vi "Periodic Tasks.vi"(8 "error in (no error)":errorcluster) -> ()   [LabVIEW 2011]
doc: "This VI runs in parallel to other tasks. It can contain as many user-defined periodic loops as you need. These can carry out PID or other sorts of timed response."
uses:
  <vilib>/Rock Robotics/SystemInterfaces/Utilities/FPGA_UtilitiesLED State.ctl
  <vilib>/Rock Robotics/SystemInterfaces/Utilities/FPGA_UtilitiesLED Source.ctl
  <vilib>/Rock Robotics/WPI/Solenoid/WPI_SolenoidValue.ctl
  <vilib>/Rock Robotics/WPI/CAN/Jaguar/SubVIs/WPI_CANJaguar_StatusSelect.ctl
  <vilib>/Rock Robotics/WPI/Compressor/WPI_CompressorGetSetRefNum.vi
  Robot Global Data.vi
  <vilib>/Rock Robotics/WPI/Solenoid/Deprecated/WPI_SolenoidGetBool.vi
  <vilib>/Rock Robotics/WPI/Solenoid/WPI_SolenoidSetEnum.vi
panel:
  out "index":i32
  out "Target Locked":bool
  out "is not locked":bool
  out "is locked":bool
  out "Actual RPM":dbl
  out "Calculated RPM":dbl
  out "small error":bool
  out "poutput":dbl
  out "Distance from dash":dbl
  out "lr-v-out":dbl
  in  "Distance":dbl
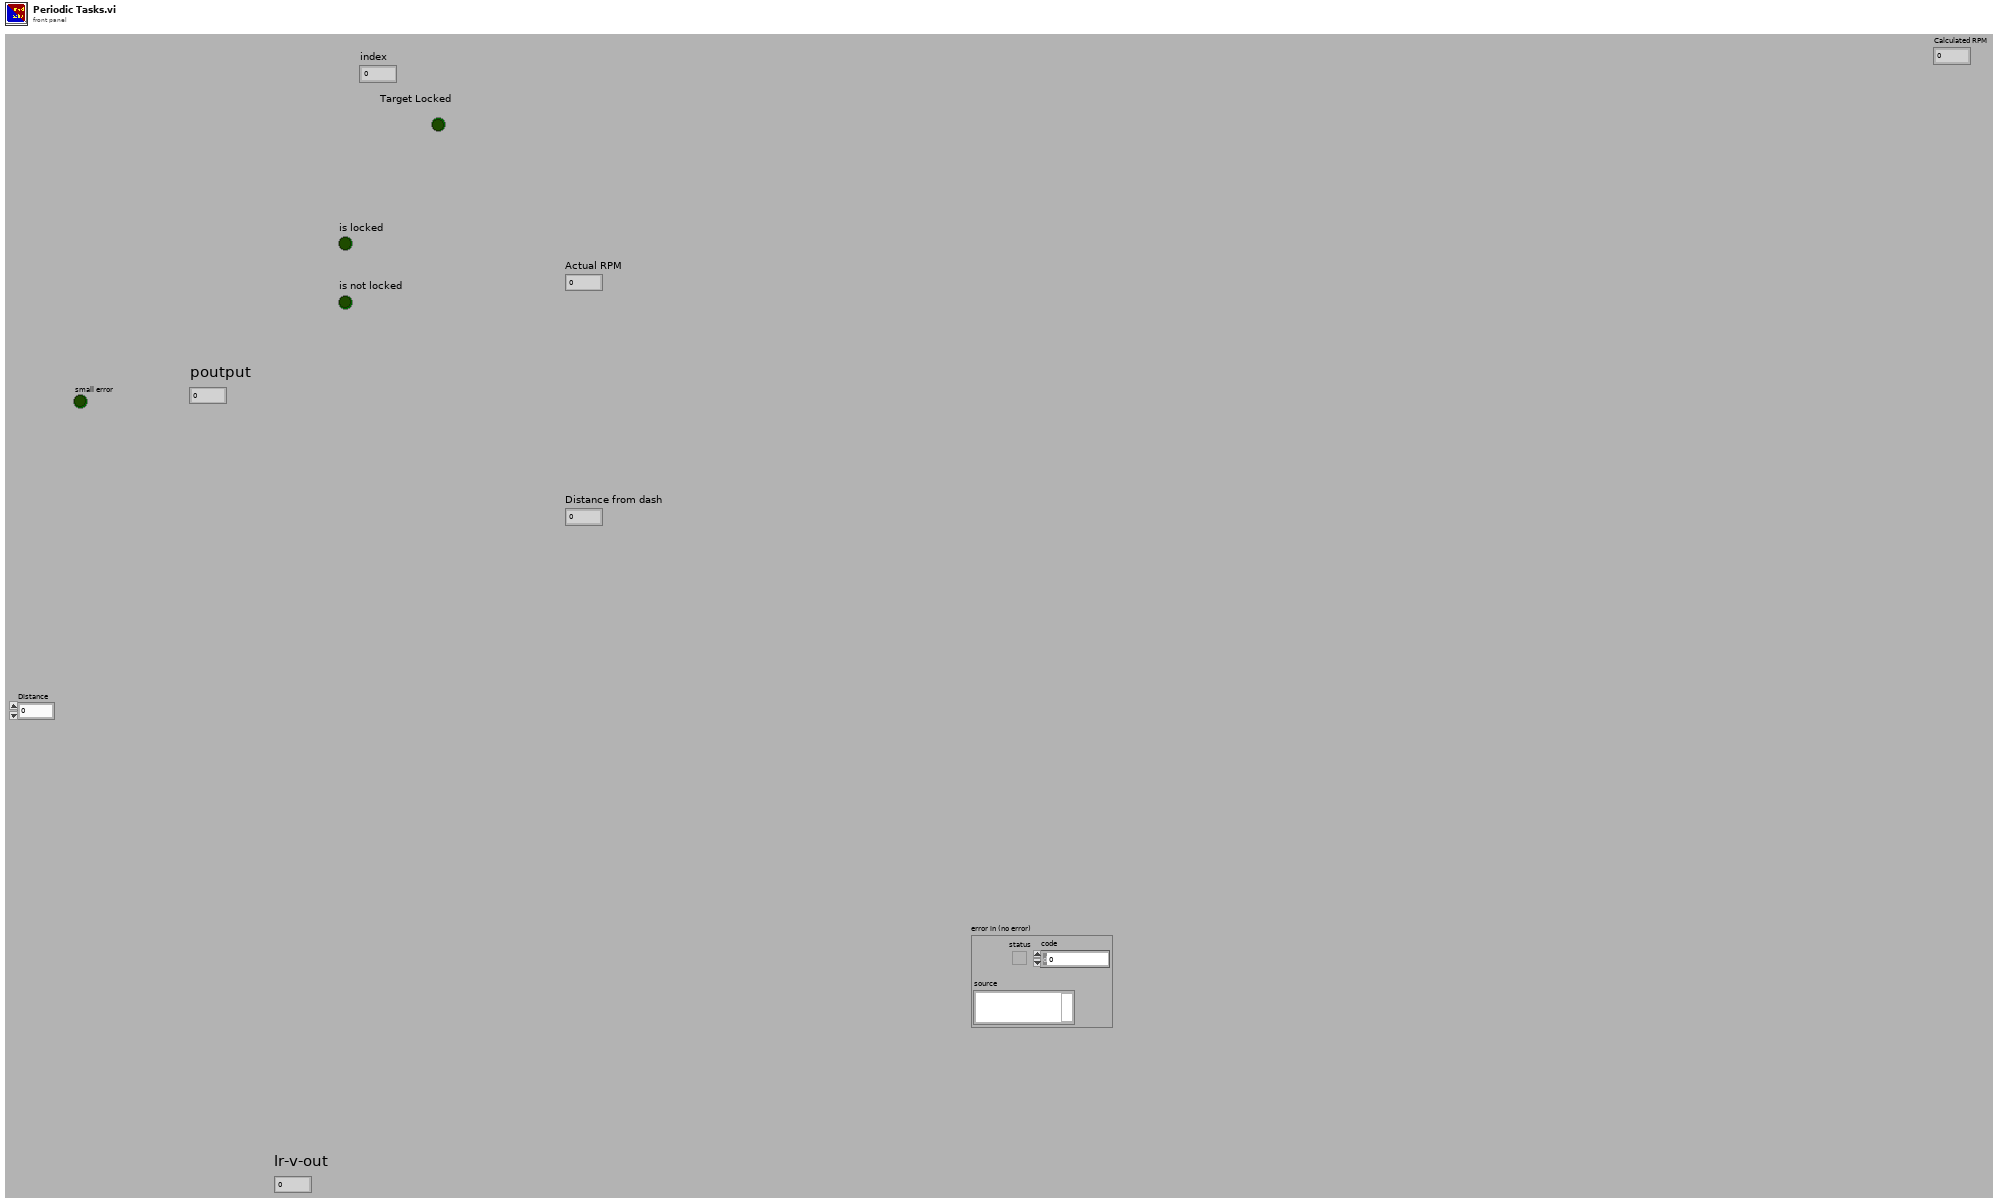
[diagram p1: front panel]
types:
  T1 = typedef "WPI_JoystickDevRef.ctl" = cluster{"Device":T2}
  T2 = typedef "WPI_JoystickDeviceEnum.ctl" = enum16{"USB 1", "USB 2", "USB 3", "USB 4", "Kinect 1", "Kinect 2"}
  T3 = typedef "WPI_JoystickButtonState.ctl" = cluster{"Button 1":bool, "Button 2":bool, "Button 3":bool, "Button 4":bool, "Button 5":bool, "Button 6":bool, "Button 7":bool, "Button 8":bool, "Button 9":bool, "Button 10":bool, "Button 11":bool, "Button 12":bool}
  T4 = cluster{"axis 1 (x)":dbl, "axis 2 (y)":dbl, "axis 3 (throttle)":dbl, "axis 4":dbl, "axis 5":dbl, "axis 6":dbl}
  T5 = typedef "WPI_CANJaguar_StatusSelect.ctl" = enum16{"Output Percent VBus", "Output Voltage", "Bus Voltage", "Current", "Temperature", "Position", "Speed", "Limit Switches", "Faults", "Fault Counters", "Power Cycle"}
  T6 = typedef "WPI_MotorControlDeviceRef.ctl" = cluster{"DeviceStatus":errorcluster, "Type":enum16{"PWM", "CAN"}, "PWM":cluster{"Digital Module":T7, "PWM Channel":T8, "DeadBand":T9}, "CAN":cluster{"Device Number":u8, "Control Mode":T10, "Semaphore":T11, "Max Vout":dbl}, "Invert":bool, "TransformRef":T12, "InvTransformRef":T12}
  T7 = typedef "FPGA_TypedefDigitalModule.ctl" = enum16{"Digital Module 1", "Digital Module 2"}
  T8 = typedef "FPGA_DIOPWMChannel.ctl" = enum8{"PWM 1", "PWM 2", "PWM 3", "PWM 4", "PWM 5", "PWM 6", "PWM 7", "PWM 8", "PWM 9", "PWM 10", "Invalid"}
  T9 = typedef "WPI_PWMDeadband.ctl" = cluster{"Name":string, "maxPositivePwm":i32, "minPositivePwm":i32, "centerPwm":i32, "maxNegativePwm":i32, "minNegativePwm":i32, "angularRange":u16}
  T10 = typedef "WPI_CANJaguar_ControlMode.ctl" = enum8{"Percent VBus", "Current", "Speed", "Position", "Voltage"}
  T11 = typedef "Semaphore RefNum" = refnum<k1>
  T12 = typedef "WPI_PWMTransform_ConPane.ctl" = refnum<vi>
  T13 = typedef "WPI_CANJaguar_Status.ctl" = cluster{"Output Percent VBus":dbl, "Output Voltage":dbl, "Bus Voltage":dbl, "Current":dbl, "Temperature":dbl, "Position":dbl, "Speed":dbl, "Limits":cluster{"Forward Limit":bool, "Reverse Limit":bool, "Forward Soft Limit":bool, "Reverse Soft Limit":bool, "Sticky Forward Limit":bool, "Sticky Reverse Limit":bool, "Sticky Forward Soft Limit":bool, "Sticky Reverse Soft Limit":bool}, "Faults":cluster{"Current Fault":bool, "Temperature Fault":bool, "Bus Voltage Fault":bool, "Gate Driver Fault":bool, "Comm Fault":bool}, "Fault Counters":cluster{"Current Faults":u8, "Temperature Faults":u8, "Bus Voltage Faults":u8, "Gate Driver Faults":u8, "Comm Faults":u8, "CAN Status":u8, "CAN RX Errors":u8, "CAN TX Errors":u8}, "Power Cycle":bool}
  T14 = typedef "FPGA_UtilitiesLED State.ctl" = enum16{"Off", "On", "Toggle"}
  T15 = typedef "FPGA_UtilitiesLED Source.ctl" = enum16{"User LED", "FPGA LED"}
  T16 = typedef "WPI_CompressorDevRef.ctl" = cluster{"DevStatus":errorcluster, "DigitalInputDevRef":T17, "RelayDevRef":T19}
  T17 = typedef "WPI_DigitalInputDevRef.ctl" = cluster{"DevStatus":errorcluster, "DIO Channel":T18, "Digital Module":T7}
  T18 = typedef "FPGA_DIOChannel.ctl" = enum8{"DIO 1", "DIO 2", "DIO 3", "DIO 4", "DIO 5", "DIO 6", "DIO 7", "DIO 8", "DIO 9", "DIO 10", "DIO 11", "DIO 12", "DIO 13", "DIO 14", "Invalid"}
  T19 = typedef "WPI_RelayDevRef.ctl" = cluster{"DevStatus":errorcluster, "Relay Channel":T20, "Digital Module":T7, "Relay Direction":T21}
  T20 = typedef "FPGA_DIORelayChannel.ctl" = enum8{"Relay 1", "Relay 2", "Relay 3", "Relay 4", "Relay 5", "Relay 6", "Relay 7", "Relay 8", "Invalid"}
  T21 = typedef "WPI_RelayDirection.ctl" = enum16{"Both directions", "Forward only", "Reverse only"}
  T22 = typedef "WPI_DigitalOutputDevRef.ctl" = cluster{"Digital Module":T7, "DIO Channel":T18, "DevStatus":errorcluster}
  T23 = cluster{"Selected Distance":dbl, "Calculated RPM":dbl, "Actual RPM":dbl, "Target Locked":bool}
  T24 = typedef "WPI_SolenoidValue.ctl" = enum16{"Off", "On", "Forward", "Reverse"}
  T25 = typedef "WPI_SolenoidDevRef.ctl" = cluster{"DevStatus":errorcluster, "Solenoid Module":T26, "Forward Solenoid Channel":T27, "Reverse Solenoid Channel":T27}
  T26 = typedef "FPGA_TypedefSolenoidModule.ctl" = enum16{"Solenoid Module 1", "Solenoid Module 2"}
  T27 = typedef "WPI_SolenoidChannel.ctl" = enum8{"Solenoid 1", "Solenoid 2", "Solenoid 3", "Solenoid 4", "Solenoid 5", "Solenoid 6", "Solenoid 7", "Solenoid 8", "Invalid"}
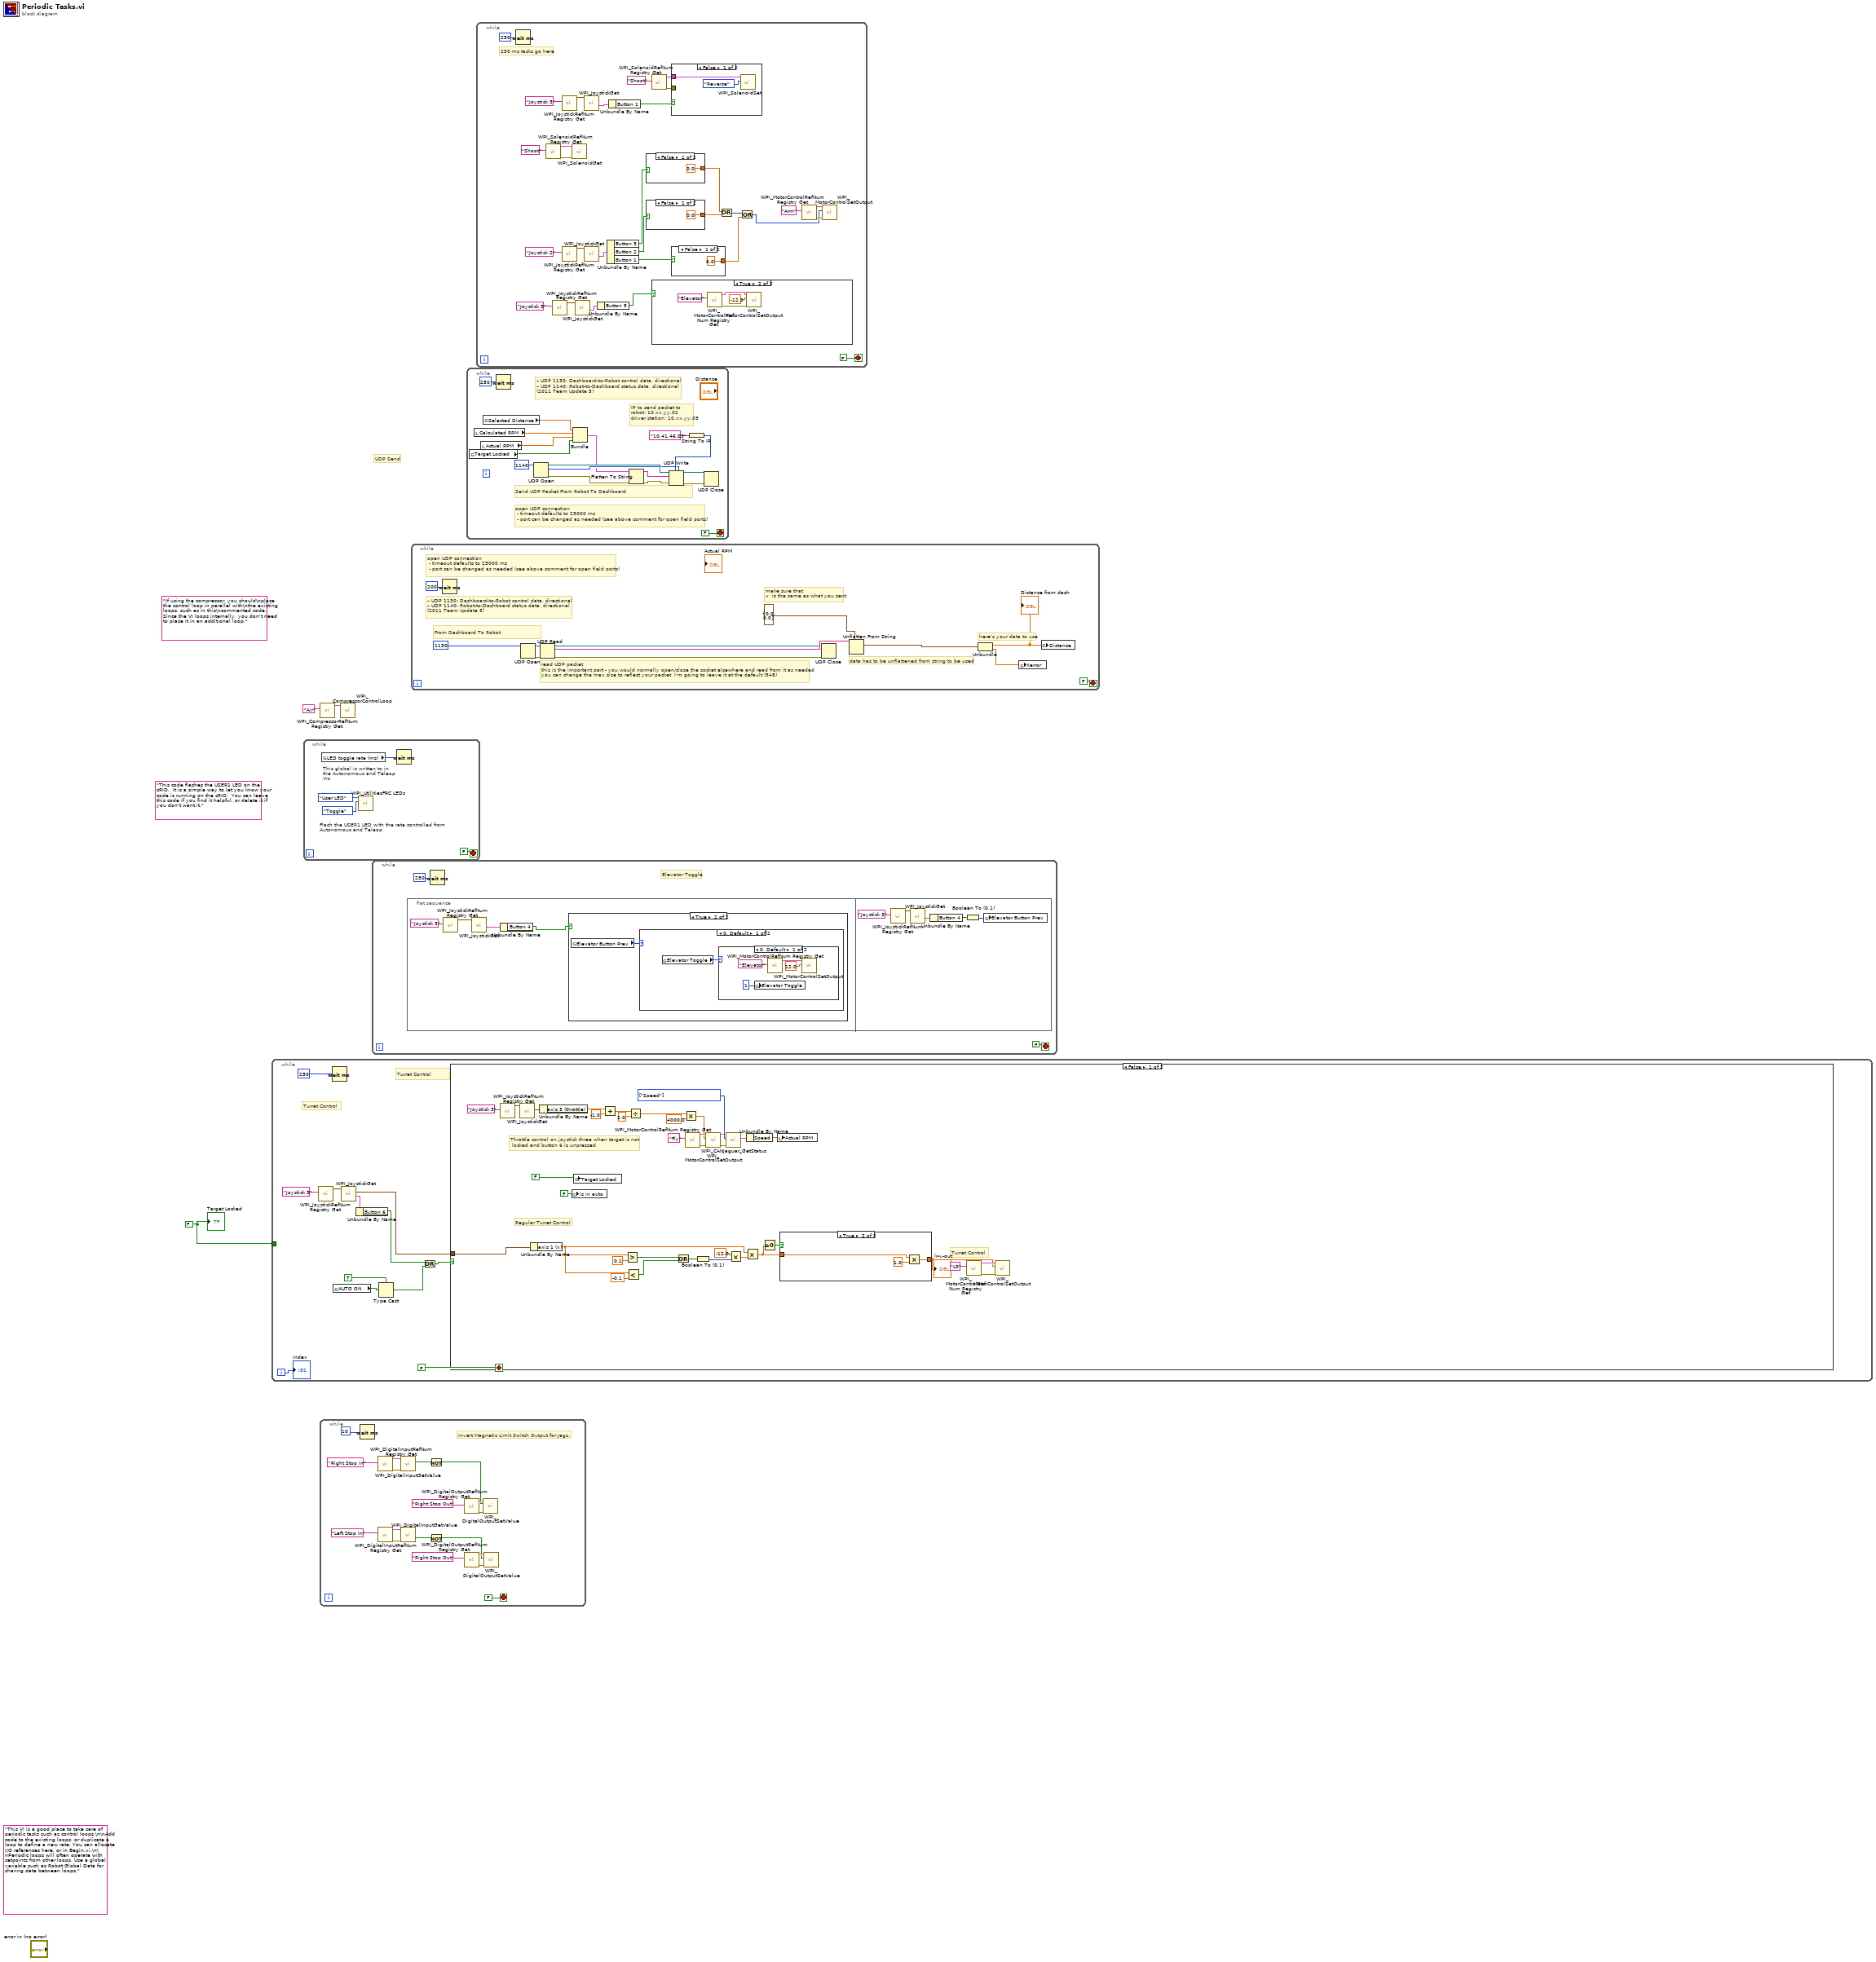
[diagram p0: block diagram]
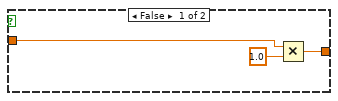
[diagram p2: hidden frame]
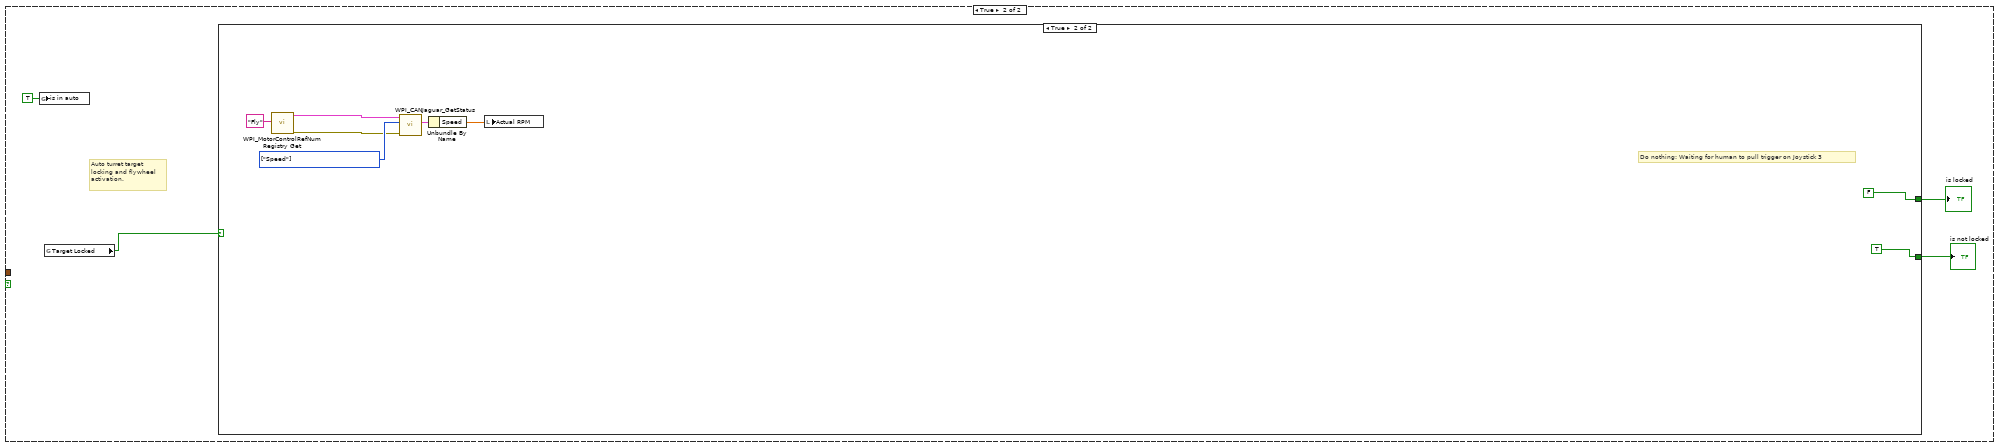
[diagram p3: hidden frame]
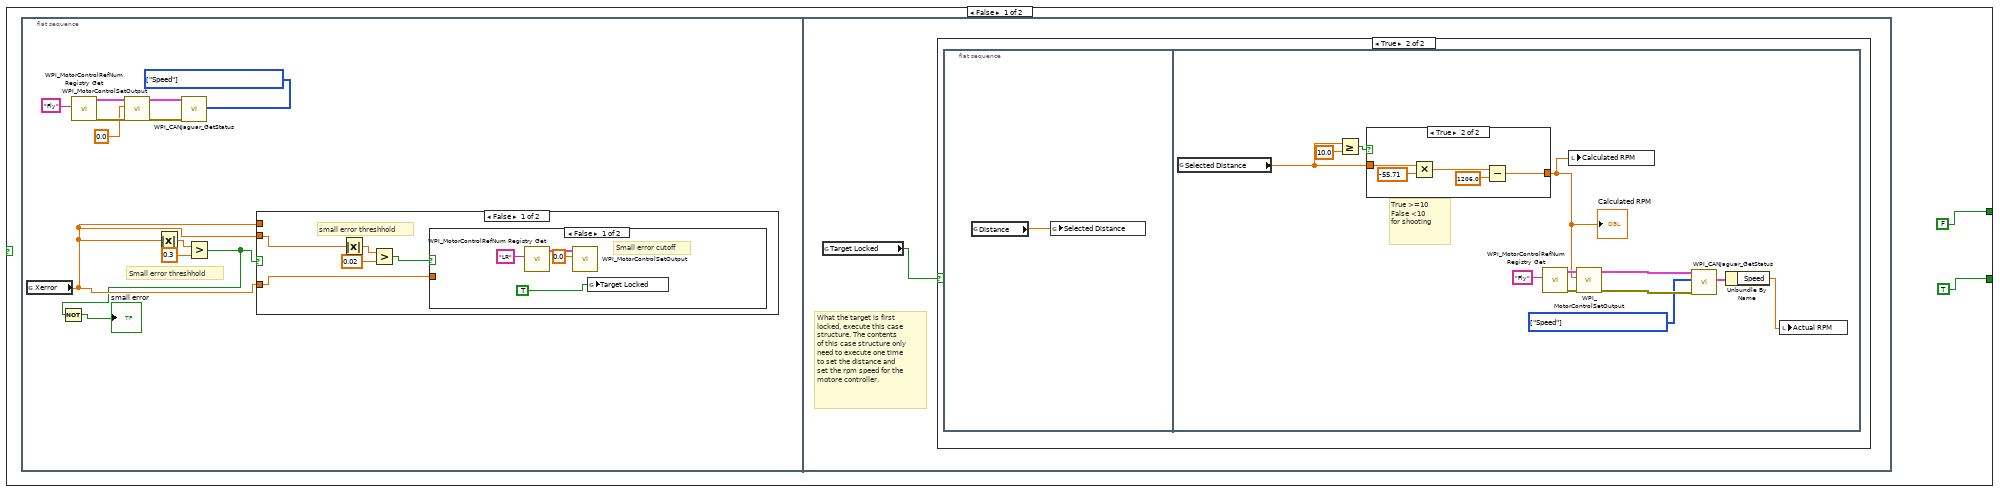
[diagram p4: hidden frame]
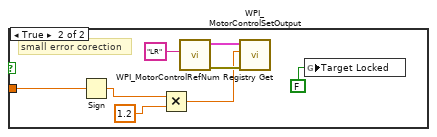
[diagram p5: hidden frame]
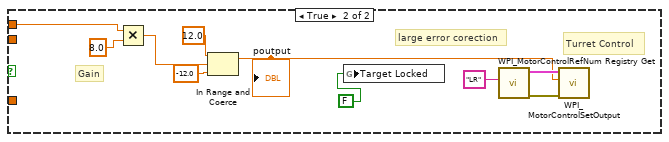
[diagram p6: hidden frame]
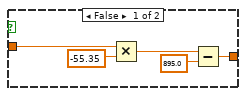
[diagram p8: hidden frame]
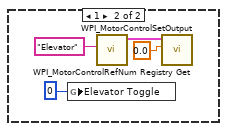
[diagram p10: hidden frame]
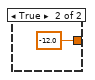
[diagram p12: hidden frame]
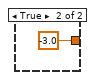
[diagram p13: hidden frame]
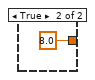
[diagram p14: hidden frame]
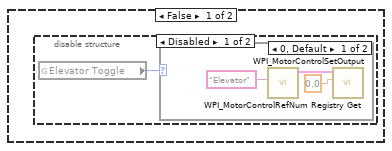
[diagram p15: hidden frame]
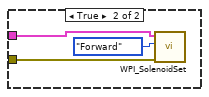
[diagram p18: hidden frame]
diagram:
  w3 = FALSE ("Target Locked")
  (unwired) "This VI is a good place to take care of periodic tasks such as control loops.\n\nAdd code to the existing loops, or duplicate a loop to define a new rate. You can allocate I/O references here, or in Begin.vi.\n\nPeriodic loops will often operate with setpoints from other loops. Use a global variable such as Robot Global Data for sharing data between loops."
  (unwired) "If using the compressor, you should\nplace the control loop in parallel with\nthe existing loops, such as in this\ncommented code. Since the VI loops internally, you don't need to place it in an additional loop."
  (unwired) "This code flashes the USER1 LED on the cRIO.  It is a simple way to let you know your code is running on the cRIO.  You can leave this code if you find it helpful, or delete it if you don't want it."
  # "UDP Send"
  n1 = while {
    tunnel: w3 -> [_]
    i -> [w10]
    stop <- FALSE stop-if-true
    # "Turret Control"
    # "Turret Control"
    n2 = call <vilib>:"WPI_JoystickRefNum Registry Get.vi"("refnum name"="Joystick 3") -> ("JoystickDevRef"=w13:T1)  [unwired: 9 in, 1 out]
    n3 = Wait (ms)(milliseconds to wait=u32 250) -> ()  [unwired: 1 out]
    n4 = global read "Robot Global Data.vi" "AUTO ON"() -> (w6:bool)
    n5 = call <vilib>:"WPI_JoystickGet.vi"("JoystickDevRef"=w13) -> ("Buttons"=w9:T3, "Axes"=w12:T4)  [unwired: 4 in, 1 out]
    n6 = Unbundle By Name(w9) -> ("Button 6"=w8:bool)
    n7 = Type Cast(type=TRUE, x=w6) -> (*(type *) &x=w4:bool)
    n8 = Or(x=w8, y=w4) -> (x .or. y?=w7:bool)
    n9 = case shown="False" w7 {
      tunnel: w12 -> [w47 _]
      frame False {
        w30 = T5[] [enum."Speed"] items=["Output Percent VBus", "Output Voltage", "Bus Voltage", "Current", "Temperature", "Position", "Speed", "Limit Switches", "Faults", "Fault Counters", "Power Cycle"] ("Status Select")
        # "Throttle control on joystick three when target is not\n locked and button 6 is unpressed"
        # "Regular Turret Control"
        # "Turret Control"
        n10 = call <vilib>:"WPI_JoystickRefNum Registry Get.vi"("refnum name"="Joystick 3") -> ("JoystickDevRef"=w26:T1)  [unwired: 9 in, 1 out]
        n11 = call <vilib>:"WPI_JoystickGet.vi"("JoystickDevRef"=w26) -> ("Axes"=w27:T4)  [unwired: 4 in, 2 out]
        n12 = Unbundle By Name(w47) -> ("axis 1 (x)"=w39:dbl)
        n13 = Unbundle By Name(w27) -> ("axis 3 (throttle)"=w24:dbl)
        n14 = global write "Robot Global Data.vi" "is in auto"(FALSE ("is in auto")) -> ()
        n15 = global write "Robot Global Data.vi" "Target Locked"(FALSE ("Target Locked")) -> ()
        n16 = Add(x=w24, y=-1.0) -> (x+y=w22:dbl)
        n17 = Greater?(x=w39, y=0.1) -> (0:w44:bool)
        n18 = Less?(x=w39, y=-0.1) -> (x < y?=w43:bool)
        n19 = Divide(x=w22, y=2.0) -> (x/y=w16:dbl)
        n20 = Or(x=w44, y=w43) -> (x .or. y?=w42:bool)
        n21 = Multiply(x=w16, y=4000.0) -> (x*y=w19:dbl)
        n22 = call <vilib>:"WPI_MotorControlRefNum Registry Get.vi"("refnum name"="Fly") -> ("error out"=w31:errorcluster, "MotorControlDevRef"=w32:T6)  [unwired: 9 in]
        n23 = Boolean To (0,1)(Boolean=w42) -> (0, 1=w41:i16)
        n24 = call <vilib>:"WPI_MotorControlSetOutput.vi"("error in (no error)"=w31, "Output"=w19, "MotorControlDevRef"=w32) -> ("error out"=w28:errorcluster, "MotorControlDevRef"=w29:T6)  [unwired: 7 in]
        n25 = call <vilib>:"WPI_CANJaguar_GetStatus.vi"("error in (no error)"=w28, "Status Select"=w30, "CAN Jaguar Ref"=w29) -> ("Status"=w18:T13)  [unwired: 6 in, 2 out]
        n26 = Multiply(x=-12.0, y=w41) -> (x*y=w40:dbl)
        n27 = Multiply(x=w39, y=w40) -> (x*y=w37:dbl)
        n28 = Unbundle By Name(w18) -> ("Speed"=w17:dbl)
        n29 = Greater Or Equal To 0?(x=w37) -> (x >= 0?=w38:bool)
        n30 = local write "Actual RPM"(w17) -> ()
        n31 = case shown="True" w38 {
          tunnel: w37 -> [w54 w57]
          tunnel: [w53 w56] -> w36
          frame False {
            n32 = Multiply(x=w54, y=1.0) -> (x*y=w53:dbl)
          }
          frame True {
            n33 = Multiply(x=w57, y=1.0) -> (x*y=w56:dbl)
          }
        }
        "lr-v-out" <- w36
        n34 = call <vilib>:"WPI_MotorControlRefNum Registry Get.vi"("refnum name"="LR") -> ("error out"=w50:errorcluster, "MotorControlDevRef"=w51:T6)  [unwired: 9 in]
        n35 = call <vilib>:"WPI_MotorControlSetOutput.vi"("error in (no error)"=w50, "Output"=w36, "MotorControlDevRef"=w51) -> ()  [unwired: 7 in, 2 out]
      }
      frame True {
        # "Auto turret target\nlocking and flywheel\nactivation."
        n36 = global write "Robot Global Data.vi" "is in auto"(TRUE ("is in auto")) -> ()
        n37 = global read "Robot Global Data.vi" "Target Locked"() -> (w58:bool)
        n38 = case shown="True" w58 {
          tunnel: [FALSE FALSE] -> w60
          tunnel: [TRUE TRUE] -> w59
          frame False {
            n39 = flat-sequence {
              frame #0 {
                w72 = T5[] [enum."Speed"] items=["Output Percent VBus", "Output Voltage", "Bus Voltage", "Current", "Temperature", "Position", "Speed", "Limit Switches", "Faults", "Fault Counters", "Power Cycle"] ("Status Select")
                # "Small error threshhold"
                n40 = global read "Robot Global Data.vi" "Xerror"() -> (w68:dbl)
                n41 = call <vilib>:"WPI_MotorControlRefNum Registry Get.vi"("refnum name"="Fly") -> ("error out"=w73:errorcluster, "MotorControlDevRef"=w74:T6)  [unwired: 9 in]
                n42 = call <vilib>:"WPI_MotorControlSetOutput.vi"("error in (no error)"=w73, "Output"=0.0, "MotorControlDevRef"=w74) -> ("error out"=w69:errorcluster, "MotorControlDevRef"=w70:T6)  [unwired: 7 in]
                n43 = Absolute Value(x=w68) -> (abs(x)=w64:dbl)
                n44 = call <vilib>:"WPI_CANJaguar_GetStatus.vi"("error in (no error)"=w69, "Status Select"=w72, "CAN Jaguar Ref"=w70) -> ()  [unwired: 6 in, 3 out]
                n45 = Greater?(x=w64, y=0.3) -> (0:w67:bool)
                n46 = Not(x=w67) -> (.not. x?=→"small error":bool)
                n47 = case shown="False" w67 {
                  tunnel: w68 -> [_ w98]
                  tunnel: w68 -> [w80 _]
                  tunnel: w68 -> [w77 _]
                  frame False {
                    # "small error threshhold"
                    n48 = Absolute Value(x=w77) -> (abs(x)=w79:dbl)
                    n49 = Greater?(x=w79, y=0.02) -> (0:w76:bool)
                    n50 = case shown="False" w76 {
                      tunnel: w80 -> [_ w89]
                      frame False {
                        # "Small error cutoff"
                        n51 = call <vilib>:"WPI_MotorControlRefNum Registry Get.vi"("refnum name"="LR") -> ("MotorControlDevRef"=w84:T6)  [unwired: 9 in, 1 out]
                        n52 = call <vilib>:"WPI_MotorControlSetOutput.vi"("Output"=0.0, "MotorControlDevRef"=w84) -> ()  [unwired: 8 in, 2 out]
                        n53 = global write "Robot Global Data.vi" "Target Locked"(TRUE ("Target Locked")) -> ()
                      }
                      frame True {
                        # "small error corection"
                        n54 = Sign(1:w89) -> (0:w88:dbl)
                        n55 = Multiply(x=w88, y=1.2) -> (x*y=w87:dbl)
                        n56 = call <vilib>:"WPI_MotorControlRefNum Registry Get.vi"("refnum name"="LR") -> ("error out"=w91:errorcluster, "MotorControlDevRef"=w92:T6)  [unwired: 9 in]
                        n57 = call <vilib>:"WPI_MotorControlSetOutput.vi"("error in (no error)"=w91, "Output"=w87, "MotorControlDevRef"=w92) -> ()  [unwired: 7 in, 2 out]
                        n58 = global write "Robot Global Data.vi" "Target Locked"(FALSE ("Target Locked")) -> ()
                      }
                    }
                  }
                  frame True {
                    # "large error corection"
                    # "Gain"
                    # "Turret Control"
                    n59 = Multiply(x=w98, y=8.0) -> (x*y=w95:dbl)
                    n60 = In Range and Coerce(upper limit=12.0, x=w95, lower limit=-12.0) -> (coerced(x)=w97:dbl)  [unwired: 1 out]
                    "poutput" <- w97
                    n61 = global write "Robot Global Data.vi" "Target Locked"(FALSE ("Target Locked")) -> ()
                    n62 = call <vilib>:"WPI_MotorControlRefNum Registry Get.vi"("refnum name"="LR") -> ("error out"=w101:errorcluster, "MotorControlDevRef"=w102:T6)  [unwired: 9 in]
                    n63 = call <vilib>:"WPI_MotorControlSetOutput.vi"("error in (no error)"=w101, "Output"=w97, "MotorControlDevRef"=w102) -> ()  [unwired: 7 in, 2 out]
                  }
                }
              }
              frame #1 {
                # "What the target is first\nlocked, execute this case\nstructure. The contents\nof this case structure only\nneed to execute one time\nto set the distance and\nset the rpm speed for the\nmotore controller."
                n64 = global read "Robot Global Data.vi" "Target Locked"() -> (w103:bool)
                n65 = case shown="True" w103 {
                  frame False {
                  }
                  frame True {
                    n66 = flat-sequence {
                      frame #0 {
                        n67 = global read "Robot Global Data.vi" "Distance"() -> (w104:dbl)
                        n68 = global write "Robot Global Data.vi" "Selected Distance"(w104) -> ()
                      }
                      frame #1 {
                        w109 = T5[] [enum."Speed"] items=["Output Percent VBus", "Output Voltage", "Bus Voltage", "Current", "Temperature", "Position", "Speed", "Limit Switches", "Faults", "Fault Counters", "Power Cycle"] ("Status Select")
                        # "True >=10\nFalse <10\nfor shooting"
                        n69 = global read "Robot Global Data.vi" "Selected Distance"() -> (w107:dbl)
                        n70 = Greater Or Equal?(x=w107, y=10.0) -> (x >= y?=w112:bool)
                        n71 = case shown="True" w112 {
                          tunnel: w107 -> [w117 w122]
                          tunnel: [w121 w126] -> w106
                          frame False {
                            n72 = Multiply(x=w117, y=-55.35) -> (x*y=w119:dbl)
                            n73 = Subtract(x=w119, y=895.0) -> (x-y=w121:dbl)
                          }
                          frame True {
                            n74 = Multiply(x=w122, y=-55.71) -> (x*y=w124:dbl)
                            n75 = Subtract(x=w124, y=1206.0) -> (x-y=w126:dbl)
                          }
                        }
                        "Calculated RPM" <- w106
                        n76 = call <vilib>:"WPI_MotorControlRefNum Registry Get.vi"("refnum name"="Fly") -> ("error out"=w114:errorcluster, "MotorControlDevRef"=w115:T6)  [unwired: 9 in]
                        n77 = local write "Calculated RPM"(w106) -> ()
                        n78 = call <vilib>:"WPI_MotorControlSetOutput.vi"("error in (no error)"=w114, "Output"=w106, "MotorControlDevRef"=w115) -> ("error out"=w110:errorcluster, "MotorControlDevRef"=w111:T6)  [unwired: 7 in]
                        n79 = call <vilib>:"WPI_CANJaguar_GetStatus.vi"("error in (no error)"=w110, "Status Select"=w109, "CAN Jaguar Ref"=w111) -> ("Status"=w108:T13)  [unwired: 6 in, 2 out]
                        n80 = Unbundle By Name(w108) -> ("Speed"=w105:dbl)
                        n81 = local write "Actual RPM"(w105) -> ()
                      }
                    }
                  }
                }
              }
            }
          }
          frame True {
            w133 = T5[] [enum."Speed"] items=["Output Percent VBus", "Output Voltage", "Bus Voltage", "Current", "Temperature", "Position", "Speed", "Limit Switches", "Faults", "Fault Counters", "Power Cycle"] ("Status Select")
            # "Do nothing: Waiting for human to pull trigger on Joystick 3"
            n82 = call <vilib>:"WPI_MotorControlRefNum Registry Get.vi"("refnum name"="Fly") -> ("error out"=w129:errorcluster, "MotorControlDevRef"=w130:T6)  [unwired: 9 in]
            n83 = call <vilib>:"WPI_CANJaguar_GetStatus.vi"("error in (no error)"=w129, "Status Select"=w133, "CAN Jaguar Ref"=w130) -> ("Status"=w132:T13)  [unwired: 6 in, 2 out]
            n84 = Unbundle By Name(w132) -> ("Speed"=w131:dbl)
            n85 = local write "Actual RPM"(w131) -> ()
          }
        }
        "is locked" <- w60
        "is not locked" <- w59
      }
    }
    "index" <- w10
  }
  n86 = while {
    stop <- FALSE stop-if-true
    # "This global is written to in the Autonomous and Teleop VIs"
    # "Flash the USER1 LED with the rate controlled from Autonomous and Teleop"
    n87 = global read "Robot Global Data.vi" "LED toggle rate (ms)"() -> (w135:u32)
    n88 = call <vilib>:"WPI_UtilitiesFRC LEDs.vi"("State"=FPGA_UtilitiesLED_State."Toggle", "LED Type"=FPGA_UtilitiesLED_Source."User LED") -> ()  [unwired: 1 in, 9 out]
    n89 = Wait (ms)(milliseconds to wait=w135) -> ()  [unwired: 1 out]
  }
  n90 = call <vilib>:"WPI_CompressorRefNum Registry Get.vi"("refnum name"="Air") -> ("CompressorDevRef"=w2:T16)  [unwired: 9 in, 1 out]
  n91 = while {
    stop <- FALSE stop-if-true
    # "Invert Magnetic Limit Switch Output for Jags."
    n92 = Wait (ms)(milliseconds to wait=u32 10) -> ()  [unwired: 1 out]
    n93 = call <vilib>:"WPI_DigitalInputRefNum Registry Get.vi"("refnum name"="Right Stop In") -> ("error out"=w149:errorcluster, "DigitalInputDevRef"=w152:T17)  [unwired: 9 in]
    n94 = call <vilib>:"WPI_DigitalInputRefNum Registry Get.vi"("refnum name"="Left Stop In") -> ("error out"=w150:errorcluster, "DigitalInputDevRef"=w153:T17)  [unwired: 9 in]
    n95 = call <vilib>:"WPI_DigitalInputGetValue.vi"("error in (no error)"=w149, "DigitalInputDevRef"=w152) -> ("Value"=w140:bool)  [unwired: 7 in, 2 out]
    n96 = call <vilib>:"WPI_DigitalInputGetValue.vi"("error in (no error)"=w150, "DigitalInputDevRef"=w153) -> ("Value"=w142:bool)  [unwired: 7 in, 2 out]
    n97 = Not(x=w140) -> (.not. x?=w139:bool)
    n98 = Not(x=w142) -> (.not. x?=w141:bool)
    n99 = call <vilib>:"WPI_DigitalOutputRefNum Registry Get.vi"("refnum name"="Right Stop Out") -> ("error out"=w144:errorcluster, "DigitalOutputDevRef"=w143:T22)  [unwired: 9 in]
    n100 = call <vilib>:"WPI_DigitalOutputRefNum Registry Get.vi"("refnum name"="Right Stop Out") -> ("error out"=w146:errorcluster, "DigitalOutputDevRef"=w145:T22)  [unwired: 9 in]
    n101 = call <vilib>:"WPI_DigitalOutputSetValue.vi"("error in (no error)"=w144, "Value"=w139, "DigitalOutputDevRef"=w143) -> ()  [unwired: 7 in, 2 out]
    n102 = call <vilib>:"WPI_DigitalOutputSetValue.vi"("error in (no error)"=w146, "Value"=w141, "DigitalOutputDevRef"=w145) -> ()  [unwired: 7 in, 2 out]
  }
  n103 = call <vilib>:"WPI_CompressorControlLoop.vi"("CompressorDevRef"=w2) -> ()  [unwired: 11 in]
  n104 = while {
    stop <- FALSE stop-if-true
    # "Elevator Toggle"
    n105 = flat-sequence {
      frame #0 {
        n106 = call <vilib>:"WPI_JoystickRefNum Registry Get.vi"("refnum name"="Joystick 3") -> ("JoystickDevRef"=w161:T1)  [unwired: 9 in, 1 out]
        n107 = call <vilib>:"WPI_JoystickGet.vi"("JoystickDevRef"=w161) -> ("Buttons"=w160:T3)  [unwired: 4 in, 2 out]
        n108 = Unbundle By Name(w160) -> ("Button 4"=w159:bool)
        n109 = case shown="True" w159 {
          frame False {
          }
          frame True {
            n110 = global read "Robot Global Data.vi" "Elevator Button Prev"() -> (w163:u8)
            n111 = case shown="0, Default" w163 {
              frame 0, Default {
                n112 = global read "Robot Global Data.vi" "Elevator Toggle"() -> (w164:u8)
                n113 = case shown="0, Default" w164 {
                  frame 0, Default {
                    n114 = global write "Robot Global Data.vi" "Elevator Toggle"(u8 1 ("Elevator Toggle")) -> ()
                    n115 = call <vilib>:"WPI_MotorControlRefNum Registry Get.vi"("refnum name"="Elevator") -> ("MotorControlDevRef"=w167:T6)  [unwired: 9 in, 1 out]
                    n116 = call <vilib>:"WPI_MotorControlSetOutput.vi"("Output"=12.0 ("y"), "MotorControlDevRef"=w167) -> ()  [unwired: 8 in, 2 out]
                  }
                  frame 1 {
                    n117 = global write "Robot Global Data.vi" "Elevator Toggle"(u8 0 ("Elevator Toggle")) -> ()
                    n118 = call <vilib>:"WPI_MotorControlRefNum Registry Get.vi"("refnum name"="Elevator") -> ("MotorControlDevRef"=w170:T6)  [unwired: 9 in, 1 out]
                    n119 = call <vilib>:"WPI_MotorControlSetOutput.vi"("Output"=0.0 ("y"), "MotorControlDevRef"=w170) -> ()  [unwired: 8 in, 2 out]
                  }
                }
              }
              frame 1 {
              }
            }
          }
        }
      }
      frame #1 {
        n120 = call <vilib>:"WPI_JoystickRefNum Registry Get.vi"("refnum name"="Joystick 3") -> ("JoystickDevRef"=w176:T1)  [unwired: 9 in, 1 out]
        n121 = call <vilib>:"WPI_JoystickGet.vi"("JoystickDevRef"=w176) -> ("Buttons"=w177:T3)  [unwired: 4 in, 2 out]
        n122 = Unbundle By Name(w177) -> ("Button 4"=w174:bool)
        n123 = Boolean To (0,1)(Boolean=w174) -> (0, 1=w173:i16)
        n124 = global write "Robot Global Data.vi" "Elevator Button Prev"(w173) -> ()
      }
    }
    n125 = Wait (ms)(milliseconds to wait=u32 250) -> ()  [unwired: 1 out]
  }
  n126 = while {
    stop <- FALSE stop-if-true
    # "here's your data to use"
    # "make sure that\nv  is the same as what you sent"
    # "data has to be unflattened from string to be used"
    # "read UDP packet\nthis is the important part - you would normally open/close the socket elsewhere and read from it as needed\nyou can change the max size to reflect your packet, I'm going to leave it at the default (548)"
    # "open UDP connection\n - timeout defaults to 25000 ms\n - port can be changed as needed (see above comment for open field ports)"
    # "– UDP 1130: Dashboard-to-Robot control data, directional\n– UDP 1140: Robot-to-Dashboard status data, directional\n(2011 Team Update 5)"
    # "From Dashboard To Robot"
    n127 = Wait (ms)(milliseconds to wait=u32 200) -> ()  [unwired: 1 out]
    n128 = UDP Open(11:u16 1130 ("port")) -> (port=w188:refnum<k16>, 0:w187:errorcluster)  [unwired: 1 in, 4 out]
    n129 = UDP Read(connection ID=w188, 8:w187) -> (data out=w186:string, error out=w182:errorcluster, 3:w183:refnum<k16>)  [unwired: 4 out]
    n130 = UDP Close(connection ID=w183, 8:w182) -> ()  [unwired: 2 out]
    n131 = Unflatten From String(type=cluster{dbl, dbl} {0.0, 0.0}, binary string=w186) -> (value=w184:cluster{dbl, dbl})  [unwired: 1 in, 4 out]
    n132 = Unbundle(w184) -> (w179:dbl, w178:dbl)
    "Distance from dash" <- w179
    n133 = global write "Robot Global Data.vi" "Xerror"(w178) -> ()
    n134 = global write "Robot Global Data.vi" "Distance"(w179) -> ()
  }
  n135 = while {
    stop <- FALSE stop-if-true
    # "IP to send packet to \nrobot: 10.xx.yy.02\ndriver station: 10.xx.yy.09"
    # "open UDP connection\n - timeout defaults to 25000 ms\n - port can be changed as needed (see above comment for open field ports)"
    # "Send UDP Packet From Robot To Dashboard"
    # "– UDP 1130: Dashboard-to-Robot control data, directional\n– UDP 1140: Robot-to-Dashboard status data, directional\n(2011 Team Update 5)"
    n136 = global read "Robot Global Data.vi" "Target Locked"() -> (w190:bool)
    n137 = local read "Calculated RPM"() -> (w194:dbl)
    n138 = local read "Actual RPM"() -> (w193:dbl)
    n139 = global read "Robot Global Data.vi" "Selected Distance"() -> (w195:dbl)
    n140 = Wait (ms)(milliseconds to wait=u32 250) -> ()  [unwired: 1 out]
    n141 = UDP Open(11:u16 1140 ("port")) -> (port=w199:refnum<k16>, 0:w197:errorcluster, 2:w198:u16)  [unwired: 1 in, 3 out]
    n142 = Bundle("Selected Distance"=w195, "Calculated RPM"=w194, "Actual RPM"=w193, "Target Locked"=w190) -> (w192:T23)  [unwired: 1 in]
    n143 = Flatten To String(anything=w192, error in (no error)=w197) -> (data string=w203:string, error out=w204:errorcluster)  [unwired: 3 out]
    n144 = String To IP(1:"10.41.46.09") -> (0:w205:u32)
    n145 = UDP Write(address=w205, port or service name=w198, connection ID=w199, data in=w203, 8:w204) -> (error out=w201:errorcluster, 3:w202:refnum<k16>)  [unwired: 1 out]
    n146 = UDP Close(connection ID=w202, 8:w201) -> ()  [unwired: 2 out]
  }
  n147 = while {
    stop <- FALSE stop-if-true
    # "250 ms tasks go here"
    n148 = Wait (ms)(milliseconds to wait=u32 250) -> ()  [unwired: 1 out]
    n149 = call <vilib>:"WPI_SolenoidRefNum Registry Get.vi"("refnum name"="Shoot") -> ("error out"=w231:errorcluster, "SolenoidDevRef"=w233:T25)  [unwired: 9 in]
    n150 = call <vilib>:"WPI_JoystickRefNum Registry Get.vi"("refnum name"="Joystick 3") -> ("JoystickDevRef"=w208:T1)  [unwired: 9 in, 1 out]
    n151 = call <vilib>:"WPI_JoystickRefNum Registry Get.vi"("refnum name"="Joystick 3") -> ("JoystickDevRef"=w229:T1)  [unwired: 9 in, 1 out]
    n152 = call <vilib>:"WPI_JoystickRefNum Registry Get.vi"("refnum name"="Joystick 2") -> ("JoystickDevRef"=w222:T1)  [unwired: 9 in, 1 out]
    n153 = call-poly <vilib>:"WPI_SolenoidGet.vi"("error in (no error)"=w231, "SolenoidDevRef"=w233) -> ()  [unwired: 7 in, 3 out]
    n154 = call <vilib>:"WPI_JoystickGet.vi"("JoystickDevRef"=w208) -> ("Buttons"=w210:T3)  [unwired: 4 in, 2 out]
    n155 = call <vilib>:"WPI_JoystickGet.vi"("JoystickDevRef"=w229) -> ("Buttons"=w228:T3)  [unwired: 4 in, 2 out]
    n156 = call <vilib>:"WPI_JoystickGet.vi"("JoystickDevRef"=w222) -> ("Buttons"=w232:T3)  [unwired: 4 in, 2 out]
    n157 = Unbundle By Name(w210) -> ("Button 5"=w207:bool)
    n158 = Unbundle By Name(w232) -> ("Button 3"=w218:bool, "Button 2"=w217:bool, "Button 1"=w216:bool)
    n159 = Unbundle By Name(w228) -> ("Button 1"=w224:bool)
    n160 = case shown="False" w218 {
      tunnel: [0.0 ("Output") 8.0 ("Output")] -> w214
      frame False {
      }
      frame True {
      }
    }
    n161 = case shown="False" w217 {
      tunnel: [0.0 ("Output") -3.0 ("Output")] -> w215
      frame False {
      }
      frame True {
      }
    }
    n162 = call <vilib>:"WPI_SolenoidRefNum Registry Get.vi"("refnum name"="Shoot") -> ("error out"=w225:errorcluster, "SolenoidDevRef"=w226:T25)  [unwired: 9 in]
    n163 = case shown="True" w207 {
      frame False {
        n164 = disable-structure shown="Disabled" {
          frame Disabled {
            n165 = global read "Robot Global Data.vi" "Elevator Toggle"() -> (w243:u8)
            n166 = case shown="0, Default" w243 {
              frame 0, Default {
                n167 = call <vilib>:"WPI_MotorControlRefNum Registry Get.vi"("refnum name"="Elevator") -> ("MotorControlDevRef"=w245:T6)  [unwired: 9 in, 1 out]
                n168 = call <vilib>:"WPI_MotorControlSetOutput.vi"("Output"=0.0 ("y"), "MotorControlDevRef"=w245) -> ()  [unwired: 8 in, 2 out]
              }
              frame 1 {
              }
            }
          }
          frame Enabled {
          }
        }
      }
      frame True {
        n169 = call <vilib>:"WPI_MotorControlRefNum Registry Get.vi"("refnum name"="Elevator") -> ("error out"=w247:errorcluster, "MotorControlDevRef"=w249:T6)  [unwired: 9 in]
        n170 = call <vilib>:"WPI_MotorControlSetOutput.vi"("error in (no error)"=w247, "Output"=-12.0 ("y"), "MotorControlDevRef"=w249) -> ()  [unwired: 7 in, 2 out]
      }
    }
    n171 = case shown="False" w224 {
      tunnel: w226 -> [w251 w254]
      tunnel: w225 -> [_ w253]
      frame False {
        n172 = call-poly <vilib>:"WPI_SolenoidSet.vi"("Value"=WPI_SolenoidValue."Reverse", "SolenoidDevRef"=w251) -> ()  [unwired: 8 in, 2 out]
      }
      frame True {
        n173 = call-poly <vilib>:"WPI_SolenoidSet.vi"("error in (no error)"=w253, "Value"=WPI_SolenoidValue."Forward", "SolenoidDevRef"=w254) -> ()  [unwired: 7 in, 2 out]
      }
    }
    n174 = case shown="False" w216 {
      tunnel: [0.0 ("Output") -12.0 ("Output")] -> w213
      frame False {
      }
      frame True {
      }
    }
    n175 = Or(x=w214, y=w215) -> (x .or. y?=w212:i32)
    n176 = Or(x=w212, y=w213) -> (x .or. y?=w211:i32)
    n177 = call <vilib>:"WPI_MotorControlRefNum Registry Get.vi"("refnum name"="Arm") -> ("error out"=w220:errorcluster, "MotorControlDevRef"=w221:T6)  [unwired: 9 in]
    n178 = call <vilib>:"WPI_MotorControlSetOutput.vi"("error in (no error)"=w220, "Output"=w211, "MotorControlDevRef"=w221) -> ()  [unwired: 7 in, 2 out]
  }
  "Target Locked" <- w3
